vi "主画面.vi"() -> ()   [LabVIEW 2016]
uses:
  <vilib>/Utility/sysdir.llb/System Directory Type.ctl
  <vilib>/Utility/config.llb/Read Key (String).vi
  <vilib>/Utility/config.llb/NI_LVConfig.lvlib
  data/FreeMem.dll
panel:
  in  "全屏":T1
  out "站点名称":string="站点名称"
  out "时间显示":string="2017-05-09 10:50:42"
  out "Version":string="Version:1.0.0"
  in  "主画面菜单":enum32{"首页", "数据查询", "运维调试", "系统设置"}(xcontrol)
  # "ESTD-XP 一体化微型水质自动监测站"
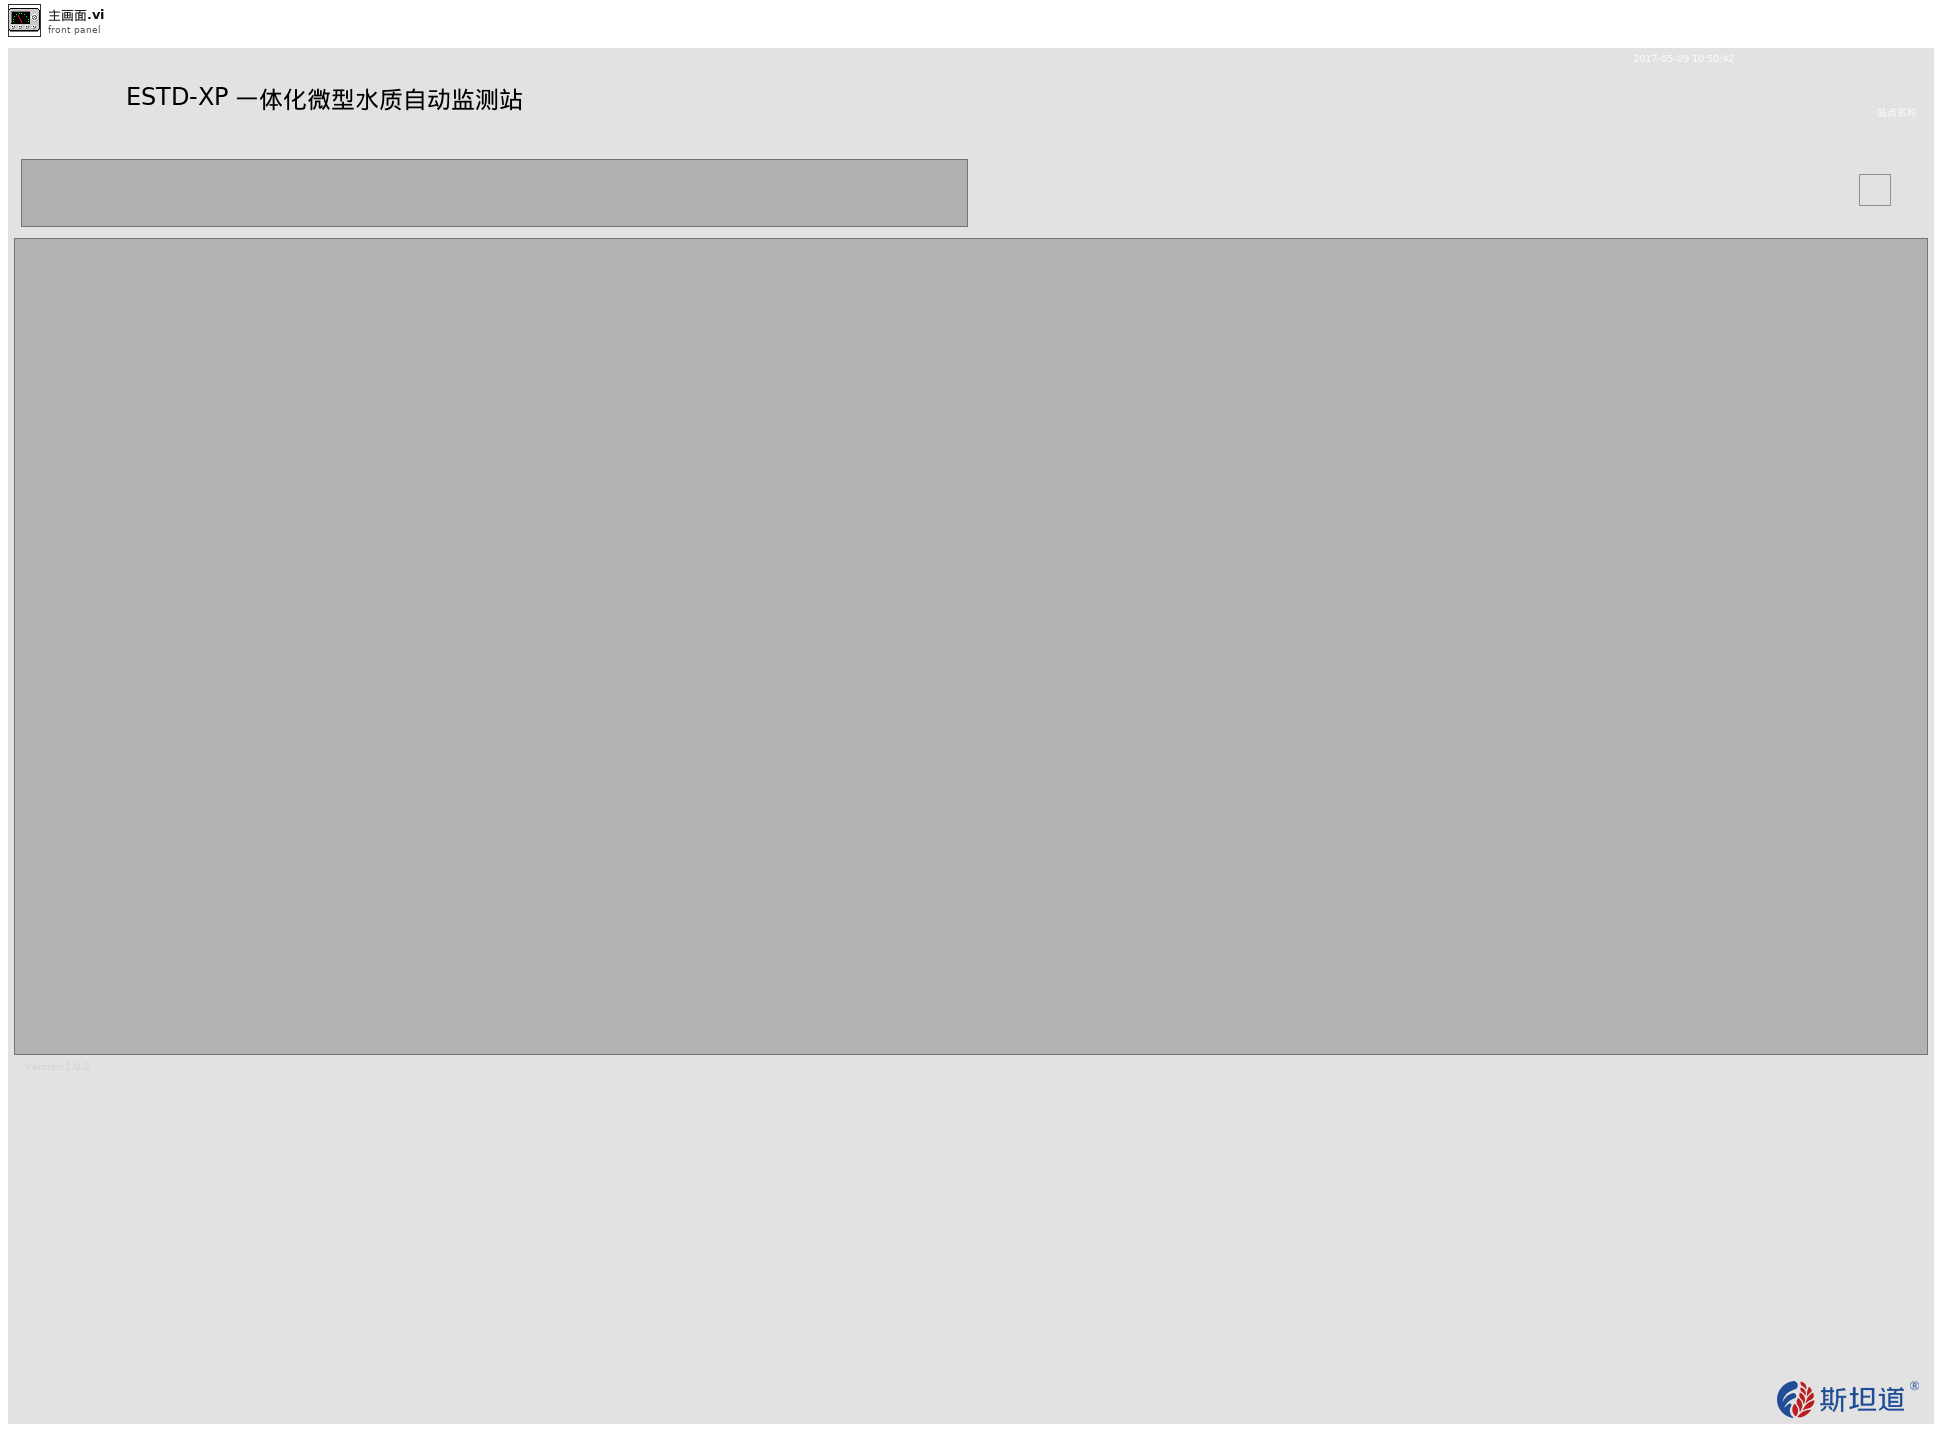
[diagram p1: front panel]
types:
  T1 = typedef "全屏按钮.ctl" = bool
  T2 = typedef "System Directory Type.ctl" = i32
  T3 = cluster{"时间标识":timestamp, "设备":string, "日志信息":string, "流程参数":string}
  T4 = enum32{"invalid app kind", "Development System", "Run Time System", "Student Edition", "Embedded LabVIEW", "Evaluation", "Custom"}
  T5 = typedef "NI_LVConfig.lvlib/Config Data RefNum.ctl" = refnum<k1>
  T6 = enum32{"Bad", "Idle", "Run top level", "Running"}
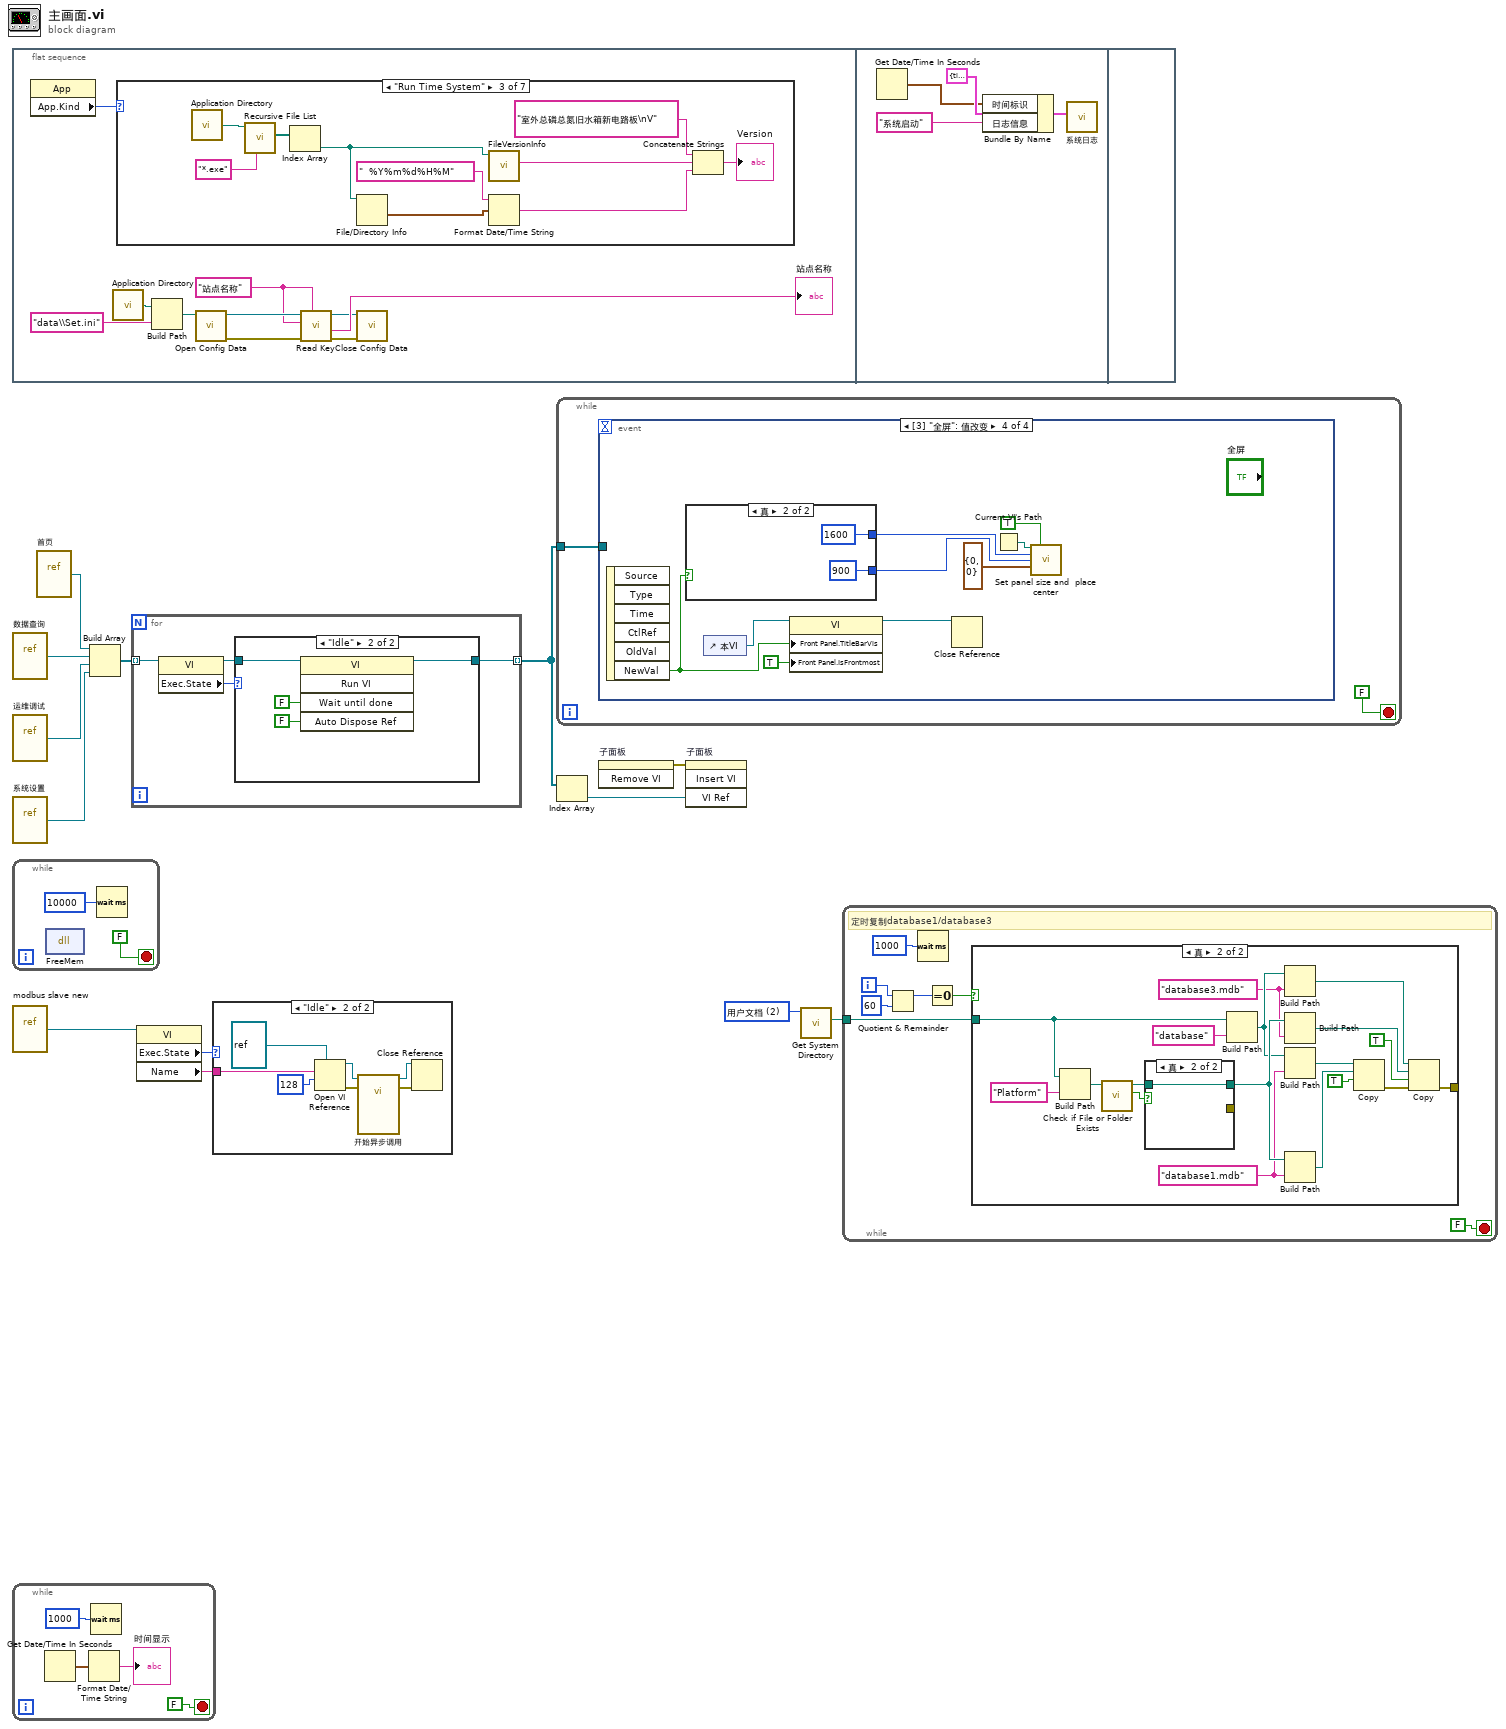
[diagram p0: block diagram]
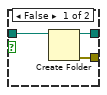
[diagram p3: hidden frame]
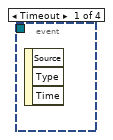
[diagram p12: hidden frame]
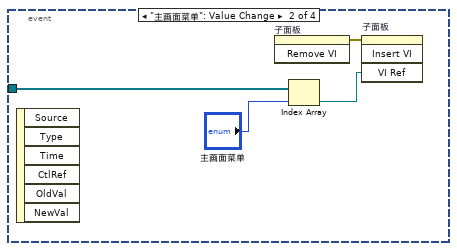
[diagram p13: hidden frame]
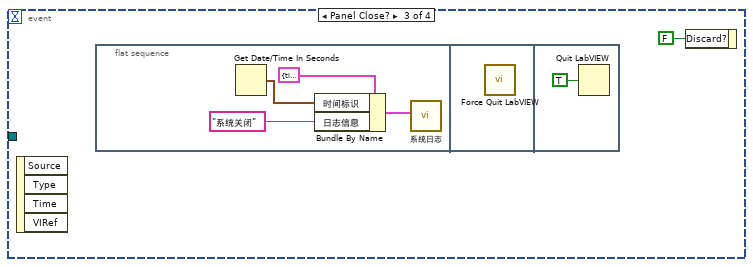
[diagram p14: hidden frame]
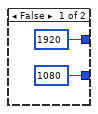
[diagram p15: hidden frame]
diagram:
  w2 = T2 2 items=["用户目录"=0, "用户桌面"=1, "用户文档"=2, "用户应用程序数据"=3, "用户设置"=4, "用户临时目录"=5, "公共文档"=6, "公共应用程序数据"=7, "公共设置"=8, "公共缓存"=13, "系统核心库"=9, "系统安装库"=10, "应用程序文件"=11, "启动盘根目录"=12] ("system directory type")
  n1 = flat-sequence {
    frame #0 {
      w14 = "站点名称" ("section")
      n2 = property class="App"() -> ("App.Kind"=w23:T4)  [unwired: 2 in, 2 out]
      n3 = call <vilib>:"Application Directory.vi"() -> ("Application Directory"=w17:path)
      n4 = case shown="\"Run Time System\"" w23 {
        frame "invalid app kind" {
        }
        frame "Development System", Default {
        }
        frame "Run Time System" {
          n5 = call <vilib>:"Application Directory.vi"() -> ("Application Directory"=w25:path)
          n6 = call <vilib>:"Recursive File List.vi"("pattern"="*.exe", "Folder Path"=w25) -> ("All Files in Dir"=w26:path[])  [unwired: 5 in, 4 out]
          n7 = Index Array(array=w26) -> (element=w24:path)  [unwired: 1 in]
          n8 = File/Directory Info(path=w24) -> (last mod=w30:timestamp)  [unwired: 1 in, 6 out]
          n9 = call <vilib>:"FileVersionInfo.vi"("Application Path in"=w24) -> ("File Version Info"=w32:string)  [unwired: 7 in, 3 out]
          n10 = Format Date/Time String(time format string (%c)="  %Y%m%d%H%M" ("时间格式字符串(%c)"), seconds (now)=w30) -> (date/time string=w28:string)  [unwired: 1 in]
          n11 = Concatenate Strings("室外总磷总氮旧水箱新电路板\nV" ("字符串"), w32, w28) -> (→"Version":string)
        }
        frame "Student Edition" {
        }
        frame "Embedded LabVIEW" {
        }
        frame "Evaluation" {
        }
        frame "Custom" {
        }
      }
      n12 = Build Path(base path=w17, name or relative path="data\\Set.ini" ("名称或相对路径")) -> (appended path=w15:path)
      n13 = call <vilib>:"Open Config Data.vi"("configuration file path"=w15) -> ("error out"=w19:errorcluster, "refnum"=w22:T5)  [unwired: 8 in, 1 out]
      n14 = call-poly <vilib>:"Read Key.vi"("section"=w14, "error in (no error)"=w19, "key"=w14, "refnum"=w22) -> ("error out"=w18:errorcluster, "value"=→"站点名称":string, "refnum out"=w20:T5)  [unwired: 4 in, 1 out]
      n15 = call <vilib>:"Close Config Data.vi"("error in (no error)"=w18, "refnum"=w20) -> ()  [unwired: 8 in, 2 out]
    }
    frame #1 {
      n16 = Get Date/Time In Seconds() -> (seconds since 1Jan1904=w35:timestamp)
      n17 = Bundle By Name(cluster=T3 {"时间标识"=timestamp(0 s since 1904-01-01), "设备"="系统", "日志信息"="", "流程参数"=""} ("data in"), "时间标识"=w35, "日志信息"="系统启动") -> (w36:T3)
      n18 = call "系统日志.vi"("data in"=w36) -> ()  [unwired: 11 in]
    }
    frame #2 {
    }
  }
  n19 = vi-ref "数据查询.vi"() -> (w9:refnum<vi>)
  n20 = vi-ref "运维调试.vi"() -> (w8:refnum<vi>)
  n21 = vi-ref "系统设置.vi"() -> (w7:refnum<vi>)
  n22 = while {
    stop <- FALSE stop-if-true
    n23 = dll-call lib="PTH2tabs CUsersHsiao\tDocumentsGIT一体站项目模板#一体站项目V2水箱新电路板dataFreeMem.dll" fn="FreeMem"() -> ()  [unwired: 4 in, 2 out]
    n24 = Wait (ms)(milliseconds to wait=u32 10000 ("等待时间（毫秒）")) -> ()  [unwired: 1 out]
  }
  n25 = vi-ref "modbus slave new.vi"() -> (w5:refnum<vi>)
  n26 = while {
    stop <- FALSE stop-if-true
    n27 = Get Date/Time In Seconds() -> (seconds since 1Jan1904=w40:timestamp)
    n28 = Format Date/Time String(seconds (now)=w40) -> (date/time string=→"时间显示":string)  [unwired: 2 in]
    n29 = Wait (ms)(milliseconds to wait=u32 1000 ("等待时间（毫秒）")) -> ()  [unwired: 1 out]
  }
  n30 = vi-ref "首页.vi"() -> (w10:refnum<vi>)
  n31 = Build Array(w10, w9, w8, w7) -> (w6:refnum<vi>[])
  n32 = for {
    tunnel: w6 -> [w47] mode=indexing
    tunnel: [w44] -> w12 mode=indexing
    n33 = property class="VI"(reference=w47) -> (reference out=w45:refnum<vi>, "Exec.State"=w46:T6)  [unwired: 1 in, 1 out]
    n34 = case shown="\"Idle\"" w46 {
      tunnel: w45 -> [w48 w50]
      tunnel: [w48 w49] -> w44
      frame "Bad", Default {
      }
      frame "Idle" {
        n35 = invoke class="VI" method="Run VI"(reference=w50, "Wait until done"=FALSE ("结束前等待"), "Auto Dispose Ref"=FALSE ("自动销毁引用")) -> (reference out=w49:refnum<vi>)  [unwired: 2 in, 4 out]
      }
    }
  }
  n36 = property class="VI"(reference=w5) -> ("Exec.State"=w4:T6, "Name"=w3:string)  [unwired: 1 in, 2 out]
  n37 = case shown="\"Idle\"" w4 {
    tunnel: w3 -> [_ w53]
    frame "Bad", Default {
    }
    frame "Idle" {
      n38 = Open VI Reference(type specifier VI Refnum (for type only)=refnum<vi> refnum, vi path=w53, options=128 ("选项")) -> (vi reference=w55:refnum<vi>, error out=w58:errorcluster)  [unwired: 3 in]
      n39 = call-by-ref "开始异步调用"(reference=w55, error in=w58) -> (reference out=w57:refnum<vi>, error out=w59:errorcluster)  [unwired: 12 in]
      n40 = Close Reference(reference=w57, error in (no error)=w59) -> ()  [unwired: 1 out]
    }
  }
  n41 = while {
    tunnel: w12 -> [w60]
    stop <- FALSE stop-if-true
    n42 = event shown="[3] \"全屏\": 值改变" {
      selector: _ -> [_ _ _ _]
      dyn-events: _ -> [_ _ _ _]
      timeout: _ -> [_ _ _ _]
      tunnel: w60 -> [_ w64 _ _]
      event Timeout {
        n43 = event-data() -> ()  [unwired: 1 in, 3 out]
      }
      event "主画面菜单": Value Change {
        n44 = event-data() -> ()  [unwired: 1 in, 6 out]
        n45 = invoke on="子面板" class="SubPnl" method="Remove VI"() -> (error out=w62:errorcluster)  [unwired: 3 in, 2 out]
        n46 = Index Array(array=w64, index="主画面菜单") -> (element=w63:refnum<vi>)
        n47 = invoke on="子面板" class="SubPnl" method="Insert VI"(error in=w62, "VI Ref"=w63) -> ()  [unwired: 2 in, 4 out]
      }
      event Panel Close? {
        n48 = event-data() -> ()  [unwired: 1 in, 4 out]
        n49 = flat-sequence {
          frame #0 {
            n50 = Get Date/Time In Seconds() -> (seconds since 1Jan1904=w69:timestamp)
            n51 = Bundle By Name(cluster=T3 {"时间标识"=timestamp(0 s since 1904-01-01), "设备"="系统", "日志信息"="", "流程参数"=""} ("data in"), "时间标识"=w69, "日志信息"="系统关闭") -> (w68:T3)
            n52 = call "系统日志.vi"("data in"=w68) -> ()  [unwired: 11 in]
          }
          frame #1 {
            n53 = call "Force Quit LabVIEW.vi"() -> ()  [unwired: 10 in, 2 out]
          }
          frame #2 {
            n54 = Quit LabVIEW(quit? (T)=TRUE ("退出？(T)")) -> ()
          }
        }
        n55 = event-data("Discard?"=FALSE ("放弃？")) -> ()  [unwired: 1 in, 1 out]
      }
      event Value Change {
        n56 = event-data() -> ("NewVal"=w75:T1)  [unwired: 1 in, 5 out]
        n57 = case shown="真" w75 {
          tunnel: [1920 ("Panel Width") 1600 ("Panel Width")] -> w74
          tunnel: [1080 ("Panel Height") 900 ("Panel Height")] -> w73
          frame False {
          }
          frame True {
          }
        }
        n58 = control-ref of="本VI"() -> (w80:refnum<vi>)
        n59 = property class="VI"(reference=w80, "Front Panel.TitleBarVis"=w75, "Front Panel.IsFrontmost"=TRUE ("前面板窗口:在最前")) -> (reference out=w76:refnum<vi>)  [unwired: 1 in, 1 out]
        n60 = Close Reference(reference=w76) -> ()  [unwired: 1 in, 1 out]
        n61 = Current VI's Path() -> (path=w79:path)
        n62 = call "Set panel size and  place center.vi"("Path"=w79, "Close Reference (false)"=TRUE, "Panel Width"=w74, "Panel Height"=w73, "FP.Origin in(H & V)"=cluster{"Horizontal":i16, "Vertical":i16} {"Horizontal"=0, "Vertical"=0}) -> ()  [unwired: 6 in, 5 out]
      }
    }
  }
  n63 = Index Array(array=w12) -> (element=w11:refnum<vi>)  [unwired: 1 in]
  n64 = invoke on="子面板" class="SubPnl" method="Remove VI"() -> (error out=w13:errorcluster)  [unwired: 3 in, 2 out]
  n65 = invoke on="子面板" class="SubPnl" method="Insert VI"(error in=w13, "VI Ref"=w11) -> ()  [unwired: 2 in, 4 out]
  n66 = call <vilib>:"Get System Directory.vi"("system directory type"=w2) -> ("system directory"=w1:path)  [unwired: 10 in]
  n67 = while {
    tunnel: w1 -> [w85]
    i -> [w89]
    stop <- FALSE stop-if-true
    # "定时复制database1/database3"
    n68 = Quotient & Remainder(x=w89, y=60) -> (x-y*floor(x/y)=w87:i32)  [unwired: 1 out]
    n69 = Wait (ms)(milliseconds to wait=u32 1000 ("等待时间（毫秒）")) -> ()  [unwired: 1 out]
    n70 = Equal To 0?(x=w87) -> (x = 0?=w86:bool)
    n71 = case shown="真" w86 {
      tunnel: w85 -> [_ w99]
      tunnel: [_ w95] -> _
      frame False {
      }
      frame True {
        w93 = "database1.mdb" ("名称或相对路径")
        w94 = "database3.mdb" ("名称或相对路径")
        n72 = Build Path(base path=w99, name or relative path="Platform" ("名称或相对路径")) -> (appended path=w106:path)
        n73 = call <vilib>:"Check if File or Folder Exists.vi"("path"=w106) -> ("file or folder exists?"=w105:bool, "dup path"=w104:path)  [unwired: 8 in, 1 out]
        n74 = case shown="真" w105 {
          tunnel: [w111 w113] -> w101
          tunnel: w104 -> [w112 w113]
          tunnel: [w110 _] -> _
          frame False {
            n75 = Create Folder(path (use dialog)=w112) -> (created path=w111:path, error out=w110:errorcluster)  [unwired: 2 in, 1 out]
          }
          frame True {
          }
        }
        n76 = Build Path(base path=w99, name or relative path="database" ("名称或相对路径")) -> (appended path=w97:path)
        n77 = Build Path(base path=w97, name or relative path=w94) -> (appended path=w96:path)
        n78 = Build Path(base path=w101, name or relative path=w94) -> (appended path=w100:path)
        n79 = Build Path(base path=w97, name or relative path=w93) -> (appended path=w98:path)
        n80 = Build Path(base path=w101, name or relative path=w93) -> (appended path=w103:path)
        n81 = Copy(9:TRUE ("覆盖(F)"), 10:w103, 11:w98) -> (0:w102:errorcluster)  [unwired: 2 in, 2 out]
        n82 = Copy(8:w102, 9:TRUE ("覆盖(F)"), 10:w100, 11:w96) -> (0:w95:errorcluster)  [unwired: 1 in, 2 out]
      }
    }
  }
